vi "Enable Frequency Correction.vi"(0 "VISA resource name":refnum<visa-resource-name>, 1 "Enable Correction (F:Disable)":bool, 5 "Frequency (100000000Hz)":dbl=100000000.0 min=-1.0 max=400000000000.0, 7 "Level (0.00dB)":dbl min=-100.0 max=100.0 format="%.3f", 11 "error in (no error)":errorcluster) -> (4 "VISA resource name out":refnum<visa-resource-name>, 15 "error out":errorcluster)   [LabVIEW 2020, in "Anritsu Signal Analyzer Series.lvlib"]
doc: "Sets whether to perform the level frequency correction processing and adds data to the level frequency correction table."
uses:
  Anritsu Signal Analyzer Series.lvlib
panel:
  # "Hz"
  # "dB"
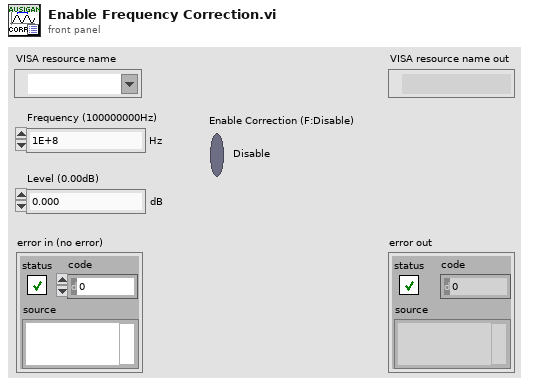
[diagram p1: front panel]
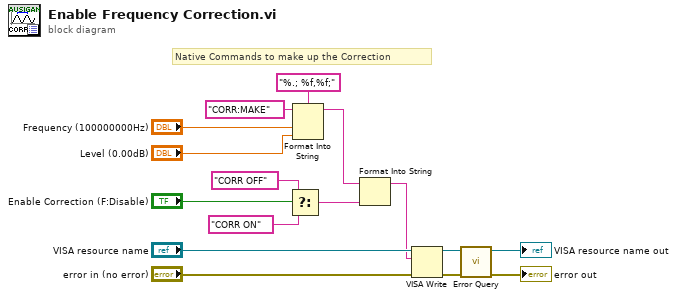
[diagram p0: block diagram]
diagram:
  # "Native Commands to make up the Correction"
  n1 = Select(t="CORR OFF", s="Enable Correction (F:Disable)", f="CORR ON") -> (s? t:f=w3:string)
  n2 = Format Into String(format string="%.; %f,%f;", initial string="CORR:MAKE" ("_Command"), "Frequency (100000000Hz)", "Level (0.00dB)") -> (resulting string=w2:string)  [unwired: 1 in, 1 out]
  n3 = Format Into String(initial string=w2, w3) -> (resulting string=w1:string)  [unwired: 2 in, 1 out]
  n4 = VISA Write(VISA resource name="VISA resource name", write buffer=w1, error in (no error)="error in (no error)") -> (VISA resource name out=w8:refnum<visa-resource-name>, error out=w7:errorcluster)  [unwired: 1 out]
  n5 = call "Error Query.vi"("error in (no error)"=w7, "VISA resource name"=w8) -> ("error out"=→"error out":errorcluster, "VISA resource name out"=→"VISA resource name out":refnum<visa-resource-name>)  [unwired: 6 in, 2 out]
